vi "Configure Reference Oscillator.vi"(6 "External Frequency (10 MHz)":dbl=10000000.0, 8 "error in (no error)":errorcluster, 9 "External Bandwidth (25 Hz)":dbl=25.0, 10 "Internal Bandwidth (25 Hz)":dbl=25.0, 11 "VISA resource name":refnum<visa-resource-name>) -> (0 "error out":errorcluster, 3 "VISA resource name out":refnum<visa-resource-name>)   [LabVIEW 2011, in "Agilent PSG MXG Series.lvlib"]
doc: "Configures internal bandwidth, external bandwidth and external frequency of the reference oscillator.\n\n<B>Notes:</B>\n(1) This VI is valid only in E8247C, E8257C, E8267C, E8257D, E8267D, N5181A, N5182A, N5183A."
uses:
  Agilent PSG MXG Series.lvlib
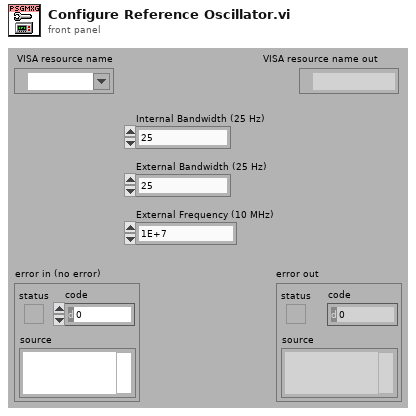
[diagram p1: front panel]
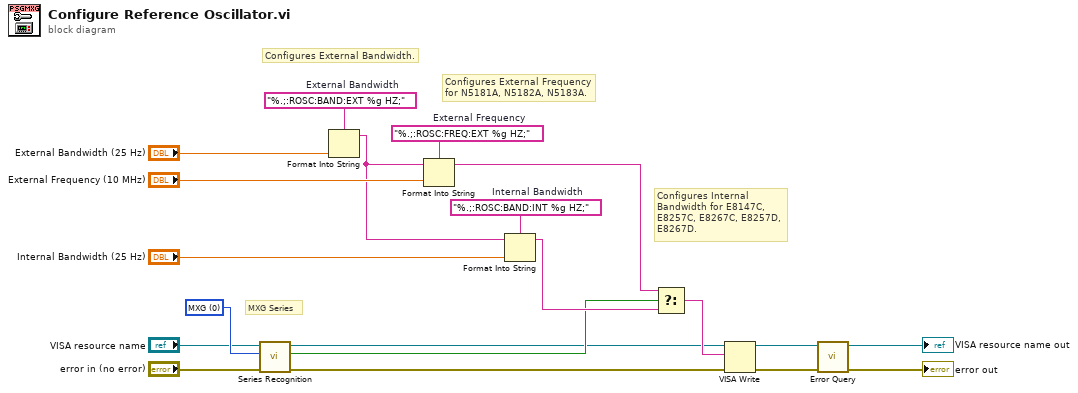
[diagram p0: block diagram]
diagram:
  w6 = u16 0 items=["MXG", "PSG", "PSG-A", "PSG-C", "PSG-D"] ("Series Type (0: MXG)")
  w16 = "%.;:ROSC:FREQ:EXT %g HZ;"  # External Frequency
  w13 = "%.;:ROSC:BAND:INT %g HZ;"  # Internal Bandwidth
  w20 = "%.;:ROSC:BAND:EXT %g HZ;"  # External Bandwidth
  # "MXG Series"
  # "Configures Internal\nBandwidth for E8147C,\nE8257C, E8267C, E8257D,\nE8267D."
  # "Configures External Frequency\nfor N5181A, N5182A, N5183A."
  # "Configures External Bandwidth."
  n1 = call "Series Recognition.vi"("error in (no error)"="error in (no error)", "Series Type (0: MXG)"=w6, "VISA resource name"="VISA resource name") -> ("error out"=w8:errorcluster, "Is Series Correct"=w7:bool, "VISA resource name out"=w5:refnum<visa-resource-name>)  [unwired: 6 in]
  n2 = Format Into String(format string=w20, "External Bandwidth (25 Hz)") -> (resulting string=w14:string)  [unwired: 2 in, 1 out]
  n3 = Format Into String(format string=w16, initial string=w14, "External Frequency (10 MHz)") -> (resulting string=w11:string)  [unwired: 1 in, 1 out]
  n4 = Format Into String(format string=w13, initial string=w14, "Internal Bandwidth (25 Hz)") -> (resulting string=w10:string)  [unwired: 1 in, 1 out]
  n5 = Select(t=w11, s=w7, f=w10) -> (s? t:f=w9:string)
  n6 = VISA Write(VISA resource name=w5, write buffer=w9, error in (no error)=w8) -> (VISA resource name out=w19:refnum<visa-resource-name>, error out=w18:errorcluster)  [unwired: 1 out]
  n7 = call "Error Query.vi"("error in (no error)"=w18, "VISA resource name"=w19) -> ("error out"=→"error out":errorcluster, "VISA resource name out"=→"VISA resource name out":refnum<visa-resource-name>)  [unwired: 6 in, 2 out]
